vi "TSM SSC Digital Get Fail Count.vi"(0 "Digital TSM In":T1, 11 "error in":errorcluster) -> (4 "Digital TSM Out":T1, 6 "Per-Site Per-Pin Fail Counts":i64[][](array[numeric]), 15 "error out":errorcluster)   [LabVIEW 2020]
doc: "Returns the per-site fail count for the specified pin(s) and pin group(s)."
uses:
  TSM/TSM SSC Digital.ctl
  <vilib>/NI_TestStand_SemiconductorModule/NI_TestStand_Semiconductor_Module.lvlibp/PinMap/Digital Pattern/PinQueryContext/DigitalPatternPinQueryContext.lvclass
  SSC Digital/SSC Digital.ctl
  be05d76c-1bdf-4e48-9376-12e4dc633cf7.vi
  Shared SubVIs/Channel List to Pins.vi
  Shared SubVIs/Trim Whitespace [Inlined].vi
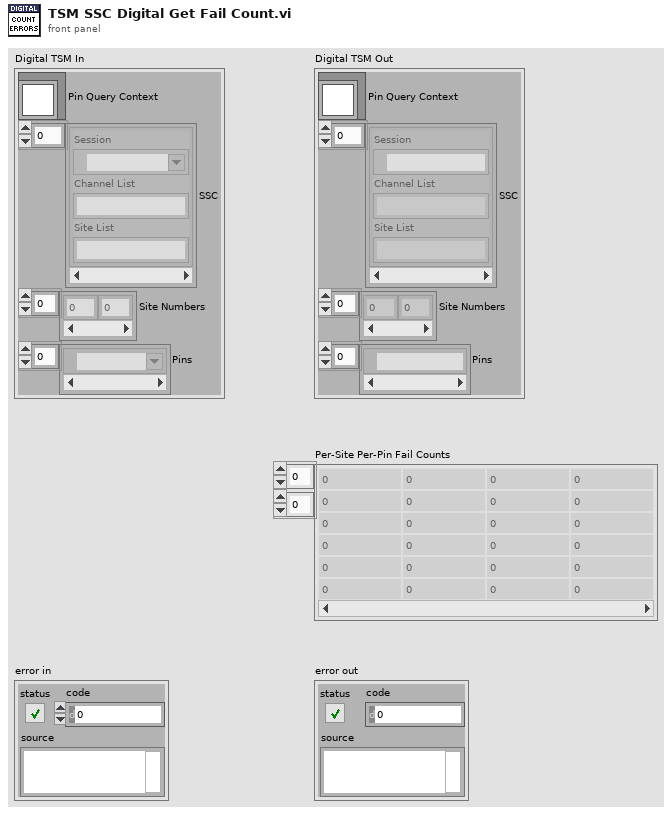
[diagram p1: front panel]
types:
  T1 = typedef "TSM SSC Digital.ctl" = cluster{"Pin Query Context":refnum<class "DigitalPatternPinQueryContext.lvclass">, "SSC":T2[], "Site Numbers":i32[], "Pins":tag[]}
  T2 = typedef "SSC Digital.ctl" = cluster{"Session":refnum<k15>, "Channel List":string, "Site List":string}
  T3 = typedef "Digital 2D Location Array in a Cluster.ctl" = cluster{"Digital 2D Location Array":T4[]}
  T4 = typedef "Digital 2D Location.ctl" = cluster{"Row":i32, "Col":i32}
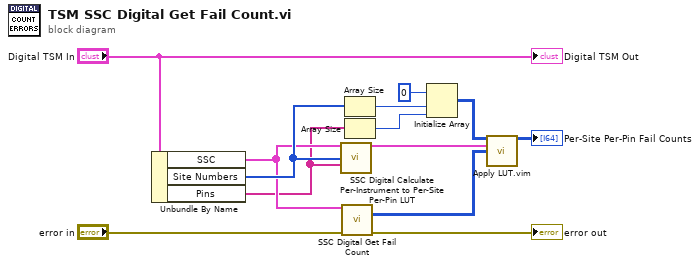
[diagram p0: block diagram]
diagram:
  n1 = Unbundle By Name("Digital TSM In") -> ("SSC"=w8:T2[], "Site Numbers"=w13:i32[], "Pins"=w6:tag[])
  n2 = call "SSC Digital Calculate Per-Instrument to Per-Site Per-Pin LUT.vi"("Digital SSC In"=w8, "Sites"=w13, "Pins"=w6) -> ("Per-Instrument to Per-Site Per-Pin LUT"=w3:T3[])  [unwired: 12 in]
  n3 = call "SSC Digital Get Fail Count.vi"("Digital SSC in"=w8, "error in"="error in") -> ("Per-Instrument Failure Counts"=w2:i64[][], "error out"=→"error out":errorcluster)  [unwired: 11 in, 1 out]
  n4 = Array Size(array=w13) -> (size(s)=w12:i32)
  n5 = Array Size(array=w6) -> (size(s)=w5:i32)
  n6 = Initialize Array(i64 0, w12, w5) -> (w4:i64[][])
  n7 = call "Apply LUT.vim"("Initialized Array"=w4, "LUT"=w3, "Results to Apply LUT to"=w2) -> ("Array Out"=→"Per-Site Per-Pin Fail Counts":i64[][])  [unwired: 12 in]
  "Digital TSM Out" <- "Digital TSM In"
